vi "check_BOP_jump.vi"(7 "Prev AO Values":fxp<+/-,20,5>[](array[numeric])=[0.0, 0.0, 0.0, 0.0, 0.0, 0.0, 0.0, 0.0, 0.0, 0.0, 0.0, 0.0, 0.0, 0.0, 0.0, 0.0], 8 "Increment Amount":fxp<+/-,20,5>, 9 "BOP jump limit":fxp<+/-,20,5>=2.0, 10 "Channel":T1={"Operation"=0, "Num. Steps"=0, "Begin"=0.0, "Step Size"=0.0, "Input - A"=0, "Input - B"=0, "Output - LO"=0.0, "Output - HI"=0.0, "Reset"=FALSE, "Analog Output"=0, "Trigger Input"=0, "Initialize To"=0, "Digital Inputs"=[0, 0, 0, 0, 0], "Output Values"=[0.0, 0.0, 0.0, 0.0, 0.0], "Num. Inputs"=4} {"Digital Inputs" items=["DIO0", "DIO1", "DIO2", "DIO3", "DIO4", "DIO5", "DIO6", "DIO7", "DIO8", "DIO9", "DIO10", "DIO11", "DIO12", "DIO13", "DIO14", "DIO15", "DIO16", "DIO17", "DIO18", "DIO19", "DIO20", "DIO21", "DIO22", "DIO23", "DIO24", "DIO25", "DIO26", "DIO27", "DIO28", "DIO29", "DIO30", "DIO31"]; "Initialize To" items=["Zero", "Begin Value"]; "Trigger Input" items=["DIO0", "DIO1", "DIO2", "DIO3", "DIO4", "DIO5", "DIO6", "DIO7", "DIO8", "DIO9", "DIO10", "DIO11", "DIO12", "DIO13", "DIO14", "DIO15", "DIO16", "DIO17", "DIO18", "DIO19", "DIO20", "DIO21", "DIO22", "DIO23", "DIO24", "DIO25", "DIO26", "DIO27", "DIO28", "DIO29", "DIO30", "DIO31"]; "Analog Output" items=["AO\\00", "AO\\01", "AO\\02", "AO\\03", "AO\\04", "AO\\05", "AO\\06", "AO\\07", "AO\\08", "AO\\09", "AO\\10", "AO\\11", "AO\\12", "AO\\13", "AO\\14", "AO\\15"]; "Input - B" items=["DIO0", "DIO1", "DIO2", "DIO3", "DIO4", "DIO5", "DIO6", "DIO7", "DIO8", "DIO9", "DIO10", "DIO11", "DIO12", "DIO13", "DIO14", "DIO15", "DIO16", "DIO17", "DIO18", "DIO19", "DIO20", "DIO21", "DIO22", "DIO23", "DIO24", "DIO25", "DIO26", "DIO27", "DIO28", "DIO29", "DIO30", "DIO31"]; "Input - A" items=["DIO0", "DIO1", "DIO2", "DIO3", "DIO4", "DIO5", "DIO6", "DIO7", "DIO8", "DIO9", "DIO10", "DIO11", "DIO12", "DIO13", "DIO14", "DIO15", "DIO16", "DIO17", "DIO18", "DIO19", "DIO20", "DIO21", "DIO22", "DIO23", "DIO24", "DIO25", "DIO26", "DIO27", "DIO28", "DIO29", "DIO30", "DIO31"]; "Operation" items=["OFF", "SWITCH", "AND GATE", "OR GATE", "ITERATION", "CUSTOM - 461nm Freq."]}, 11 "AO to Check":fxp<+/-,20,5>) -> (3 "AO Out":fxp<+/-,20,5>)   [LabVIEW 2016]
uses:
  fpga_array_element.ctl
panel:
  # "Boolean Operation Controls"
  # "Iteration Operation Controls"
  # "Custom Operation Controls"
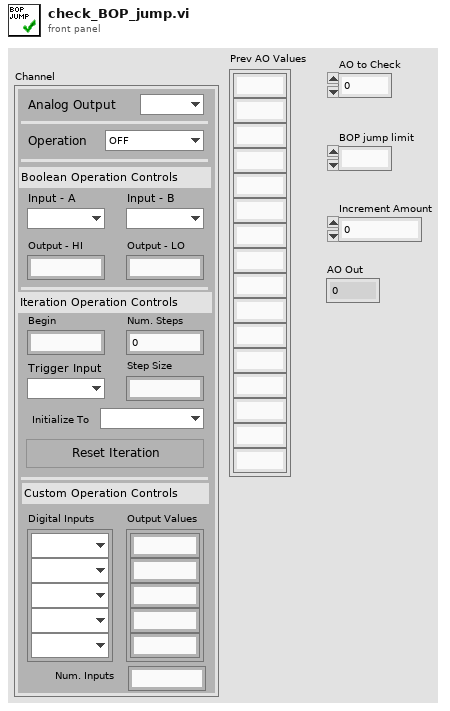
[diagram p1: front panel]
types:
  T1 = typedef "fpga_array_element.ctl" = cluster{"Operation":i16, "Num. Steps":u16, "Begin":fxp<+/-,20,5>, "Step Size":fxp<+/-,20,5>, "Input - A":i32, "Input - B":i32, "Output - LO":fxp<+/-,20,5>, "Output - HI":fxp<+/-,20,5>, "Reset":bool, "Analog Output":i32, "Trigger Input":i32, "Initialize To":i16, "Digital Inputs":i32[], "Output Values":fxp<+/-,20,5>[], "Num. Inputs":u16}
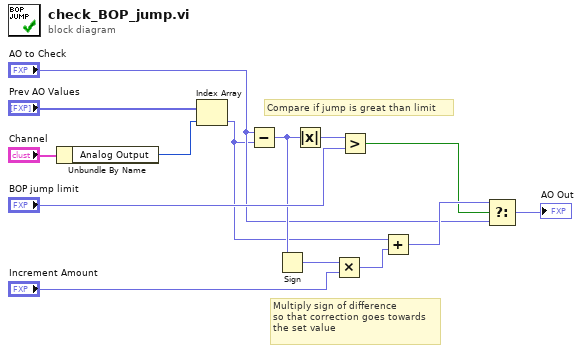
[diagram p0: block diagram]
diagram:
  # "Compare if jump is great than limit"
  # "Multiply sign of difference \nso that correction goes towards\nthe set value"
  n1 = Unbundle By Name("Channel") -> ("Analog Output"=w12:i32)
  n2 = Index Array(array="Prev AO Values", index=w12) -> (element=w1:fxp<+/-,20,5>)
  n3 = Subtract(x="AO to Check", y=w1) -> (x-y=w5:fxp<+/-,21,6>)
  n4 = Sign(1:w5) -> (0:w3:fxp<+/-,2,2>)
  n5 = Absolute Value(x=w5) -> (abs(x)=w11:fxp<+,20,5>)
  n6 = Multiply(x=w3, y="Increment Amount") -> (x*y=w4:fxp<+/-,21,6>)
  n7 = Greater?(x=w11, y="BOP jump limit") -> (0:w8:bool)
  n8 = Add(x=w1, y=w4) -> (x+y=w9:fxp<+/-,21,6>)
  n9 = Select(t=w9, s=w8, f="AO to Check") -> (s? t:f=→"AO Out":fxp<+/-,21,6>)
